vi "CleanUp.vi"(0 "object in":refnum<class "NewTestTactic.lvclass">, 5 "error in (no error)":errorcluster) -> (14 "object out":refnum<class "NewTestTactic.lvclass">, 19 "error out":errorcluster)   [LabVIEW 2022 SP3, in "NewTestTactic.lvclass"]
uses:
  NewTestTactic.lvclass
  Tactic_class/Tactic.lvclass
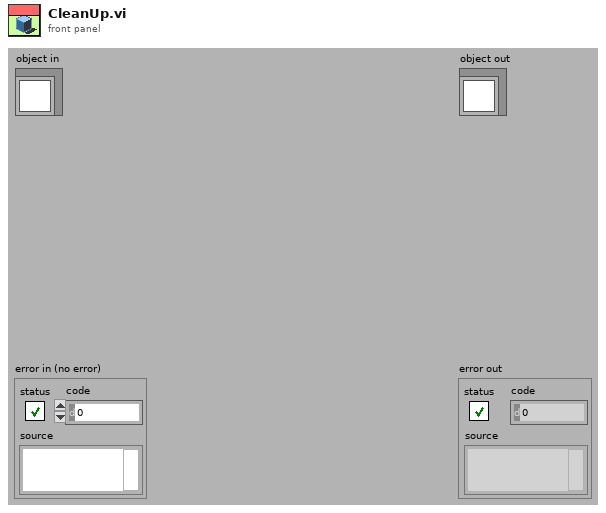
[diagram p1: front panel]
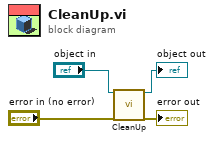
[diagram p0: block diagram]
diagram:
  n1 = call-parent "CleanUp.vi"("object in"="object in", "error in (no error)"="error in (no error)") -> ("object out"=→"object out":refnum<class "NewTestTactic.lvclass">, "error out"=→"error out":errorcluster)  [unwired: 16 in]
